vi "Setup Example All Devices.vi"(8 "error in (no error)":errorcluster, 11 "show ICL for debugging":bool) -> (0 "error out":errorcluster, 1 "Mono out":refnum<class "Monochromator.lvclass">, 2 "Module Was Already Running?":bool, 3 "CCD out":refnum<class "CCD.lvclass">, 4 "SCD out":refnum<class "SCD.lvclass">)   [LabVIEW 2020, in "Examples.lvlib"]
doc: "Setup of devices for example code execution."
uses:
  Examples/Examples.lvlib
  CCD.lvclass
  Mono/Monochromator.lvclass
  SCD/SCD.lvclass
  DeviceManager/DeviceManager.lvlib
panel:
  # "Connector Pane"
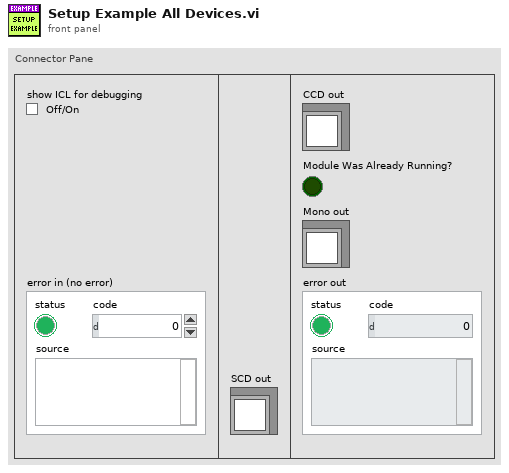
[diagram p1: front panel]
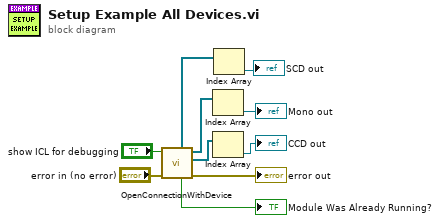
[diagram p0: block diagram]
diagram:
  n1 = call "OpenConnectionWithDevice.vi"("error in"="error in (no error)", "show ICL for debugging"="show ICL for debugging") -> ("error out"=→"error out":errorcluster, "CCDs"=w6:refnum<class "CCD.lvclass">[], "Monos"=w5:refnum<class "Monochromator.lvclass">[], "Module Was Already Running?"=→"Module Was Already Running?":bool, "SCDs"=w3:refnum<class "SCD.lvclass">[])  [unwired: 5 in]
  n2 = Index Array(array=w5) -> (element=→"Mono out":refnum<class "Monochromator.lvclass">)  [unwired: 1 in]
  n3 = Index Array(array=w6) -> (element=→"CCD out":refnum<class "CCD.lvclass">)  [unwired: 1 in]
  n4 = Index Array(array=w3) -> (element=→"SCD out":refnum<class "SCD.lvclass">)  [unwired: 1 in]
